vi "Persist Entity.vi"(8 "error in (no error)":errorcluster, 10 "Conditum:Entity":refnum<class "Entity.lvclass">, 11 "Entity Manager in":refnum<class "Entity Manager.lvclass">) -> (0 "error out":errorcluster, 3 "Entity Manager out":refnum<class "Entity Manager.lvclass">)   [LabVIEW 2020, in "Conditu2.lvlib" / "Entity Manager.lvclass"]
uses:
  Entity Manager.lvclass
  Entity/Entity.lvclass
  Entity Manager.lvclass/Entity Manager.ctl
  Database Platform/Check Relations.vi
  Columns/Relation/Validate Persistance.vi
  Columns/Relation/Relation.lvclass
  Database Platform/Database Platform.lvclass
  Unit Of Work Session/Unit Of Work Session.lvclass
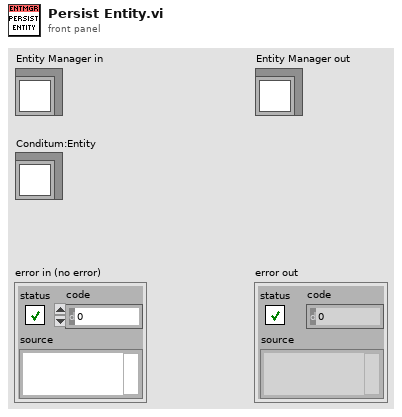
[diagram p1: front panel]
types:
  T1 = typedef "Conditu2.lvlib/Entity Manager.lvclass/Entity Info.ctl" = cluster{"Entity":refnum<class "Entity.lvclass">, "Types":refnum<class "Type.lvclass">[], "Type Name Map":map{string, i32}, "Has Relation":bool}
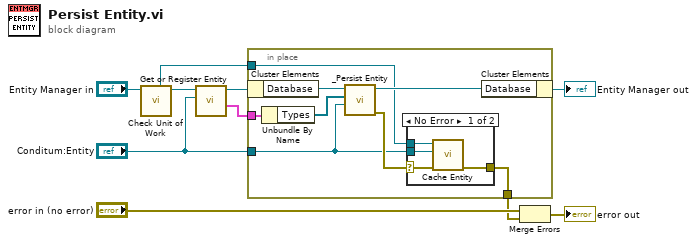
[diagram p0: block diagram]
diagram:
  n1 = call "Check Unit of Work.vi"("Entity Manager in"="Entity Manager in") -> ("Entity Manager out"=w2:refnum<class "Entity Manager.lvclass">, "Unit Of Work"=w1:refnum<class "Unit Of Work Session.lvclass">)  [unwired: 8 in, 1 out]
  n2 = call "Get or Register Entity.vi"("Entity"="Conditum:Entity", "Entity Manager in"=w2) -> ("Entity Info"=w4:T1, "Entity Manager out"=w5:refnum<class "Entity Manager.lvclass">)  [unwired: 7 in, 1 out]
  n3 = in-place {
    in-place-border: "Conditum:Entity" -> [w13]
    in-place-border: [w11] -> w7
    in-place-border: w4 -> [w16]
    in-place-border: w1 -> [w12]
    n4 = in-place-cluster #1(w5) -> ("Database"=w18:refnum<class "Database Platform.lvclass">)
    n5 = Unbundle By Name(w16) -> ("Types"=w15:refnum<class "Type.lvclass">[])
    n6 = call "_Persist Entity.vi"("Entity"=w13, "Types"=w15, "Database in"=w18) -> ("error out"=w14:errorcluster, "Database out"=w17:refnum<class "Database Platform.lvclass">)  [unwired: 7 in]
    n7 = case shown="No Error" w14 {
      selector: w14 -> [w21 w23]
      tunnel: w13 -> [w22 _]
      tunnel: w12 -> [w20 _]
      tunnel: [w19 w23] -> w11
      frame No Error {
        n8 = call "Cache Entity.vi"("error in (no error)"=w21, "Conditum:Entity"=w22, "Unit Of Work in"=w20) -> ("error out"=w19:errorcluster)  [unwired: 8 in]
      }
      frame Error {
      }
    }
    n9 = in-place-cluster #1("Database"=w17) -> (→"Entity Manager out":refnum<class "Entity Manager.lvclass">)
  }
  n10 = Merge Errors("error in (no error)", w7) -> (→"error out":errorcluster)
